vi "GetControlsFromTabPages.vi"(10 "Pages to search":string[](array[string]), 11 "Tab Control":refnum<vi>) -> (3 "Controls found":refnum<vi>[](array[refnum]))   [LabVIEW 2017]
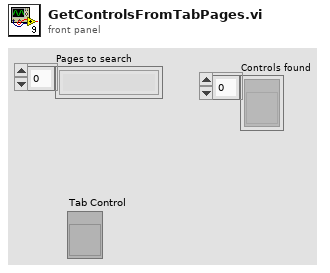
[diagram p1: front panel]
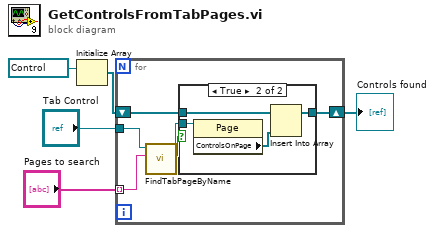
[diagram p0: block diagram]
diagram:
  n1 = Initialize Array(refnum<vi> refnum ("element")) -> (w4:refnum<vi>[])  [unwired: 1 in]
  n2 = for {
    tunnel: "Pages to search" -> [w11] mode=indexing
    shift-right: [w7] -> w2
    shift-left: w4 -> [w8]
    tunnel: "Tab Control" -> [w6]
    n3 = call "FindTabPageByName.vi"("Name"=w11, "Tab Control"=w6) -> ("found?"=w9:bool, "Page Refnum"=w10:refnum<vi>)  [unwired: 8 in]
    n4 = case shown="True" w9 {
      tunnel: w10 -> [_ w16]
      tunnel: w8 -> [w12 w15]
      tunnel: [w12 w13] -> w7
      frame False {
      }
      frame True {
        n5 = property class="Page"(reference=w16) -> ("ControlsOnPage"=w14:refnum<vi>[])  [unwired: 1 in, 2 out]
        n6 = Insert Into Array(array=w15, new element=w14) -> (w13:refnum<vi>[])  [unwired: 1 in]
      }
    }
  }
  "Controls found" <- w2
